vi "SlewRateLimiter_Calculate.vi"(8 "Time":dbl=-1.0 format="%33.4f", 9 "Input":dbl, 11 "in SLEW_RATE_LIMITER":T1 {"NegativeRateLimit" format="%13.5p"; "PrevTime" format="%30.5p"; "PrevValue" format="%13.5p"; "PositiveRateLimit" format="%13.5p"}) -> (1 "Output":dbl, 3 "out SLEW_RATE_LIMITER":T1 {"NegativeRateLimit" format="%13.5p"; "PrevTime" format="%30.5p"; "PrevValue" format="%13.5p"; "PositiveRateLimit" format="%13.5p"})   [LabVIEW 2019, in "Trajectory_Library.lvlib"]
doc: "Filters the input to limit its slew rate.\n \nInputs: \n - in Slew Rate Limiter -- The Slew Rate Limiter data cluster\n - input -- The input value whose slew rate is to be limited.\n\nOutputs:\n - out Slew Rate Limiter -- The modified Slew Rate Limiter data cluster\n - output -- The filtered value, which will not change faster than the slew rate."
uses:
  Trajectory_Library.lvlib
  TypeDef/SLEW_RATE_LIMITER.ctl
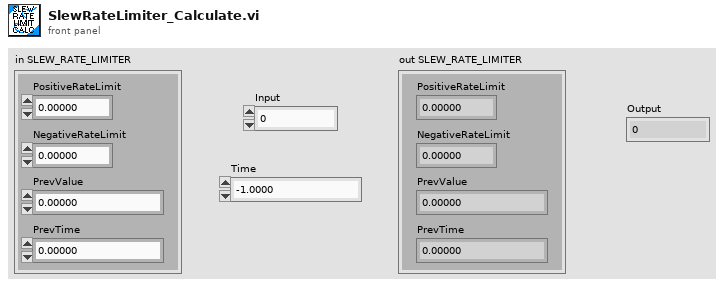
[diagram p1: front panel]
types:
  T1 = typedef "Trajectory_Library.lvlib/SLEW_RATE_LIMITER.ctl" = cluster{"PositiveRateLimit":dbl, "PrevValue":dbl, "PrevTime":dbl, "NegativeRateLimit":dbl}
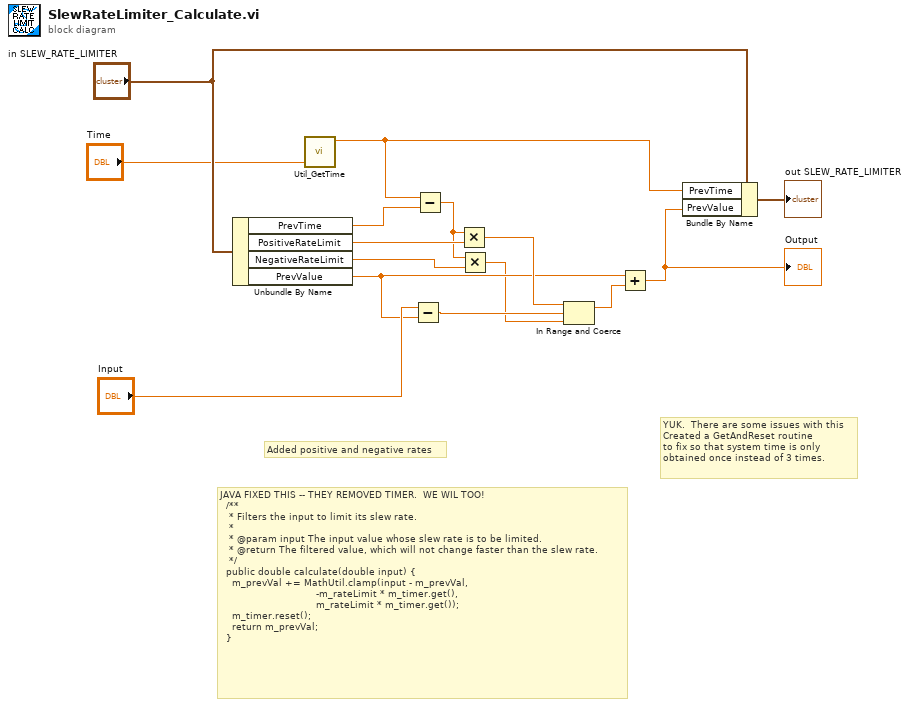
[diagram p0: block diagram]
diagram:
  # "Added positive and negative rates"
  # "YUK.  There are some issues with this\nCreated a GetAndReset routine\nto fix so that system time is only\nobtained once instead of 3 times."
  # "JAVA FIXED THIS -- THEY REMOVED TIMER.  WE WIL TOO!\n  /**\n   * Filters the input to limit its slew rate.\n   *\n   * @param input The input value whose slew rate is to be limited.\n   * @return The filtered value, which will not change faster than the slew rate.\n   */\n  public double calculate(double input) {\n    m_prevVal += MathUtil.clamp(input - m_prevVal,\n                                -m_rateLimit * m_timer.get(),\n                                m_rateLimit * m_timer.get());\n    m_timer.reset();\n    return m_prevVal;\n  }"
  n1 = Unbundle By Name("in SLEW_RATE_LIMITER") -> ("PrevTime"=w7:dbl, "PositiveRateLimit"=w13:dbl, "NegativeRateLimit"=w2:dbl, "PrevValue"=w4:dbl)
  n2 = call "Util_GetTime.vi"("Pass_Through_Time"="Time") -> ("FPGA_Time_Seconds"=w6:dbl)  [unwired: 9 in, 1 out]
  n3 = Subtract(x="Input", y=w4) -> (x-y=w10:dbl)
  n4 = Subtract(x=w6, y=w7) -> (x-y=w3:dbl)
  n5 = Multiply(x=w3, y=w13) -> (x*y=w12:dbl)
  n6 = Multiply(x=w3, y=w2) -> (x*y=w1:dbl)
  n7 = In Range and Coerce(upper limit=w12, x=w10, lower limit=w1) -> (coerced(x)=w9:dbl)  [unwired: 1 out]
  n8 = Add(x=w4, y=w9) -> (x+y=w8:dbl)
  "Output" <- w8
  n9 = Bundle By Name(cluster="in SLEW_RATE_LIMITER", "PrevTime"=w6, "PrevValue"=w8) -> (→"out SLEW_RATE_LIMITER":T1)
